vi "WriteCartesianPositionRegister.vi"(8 "Cartesian position":T1, 9 "index":i32, 10 "Snpx":refnum<k24>, 11 "error in":errorcluster) -> (3 "error out":errorcluster)   [LabVIEW 2016, in "UnderAutomation.Fanuc.lvlib"]
uses:
  UnderAutomation.Fanuc.lvlib
  C:/Users/fg/Documents/Fanuc.vi/LabVIEW_2024/UnderAutomation.Fanuc/lib/UnderAutomation.Fanuc.dll
  LabVIEW_2024/UnderAutomation.Fanuc/lib/UnderAutomation.Fanuc.dll
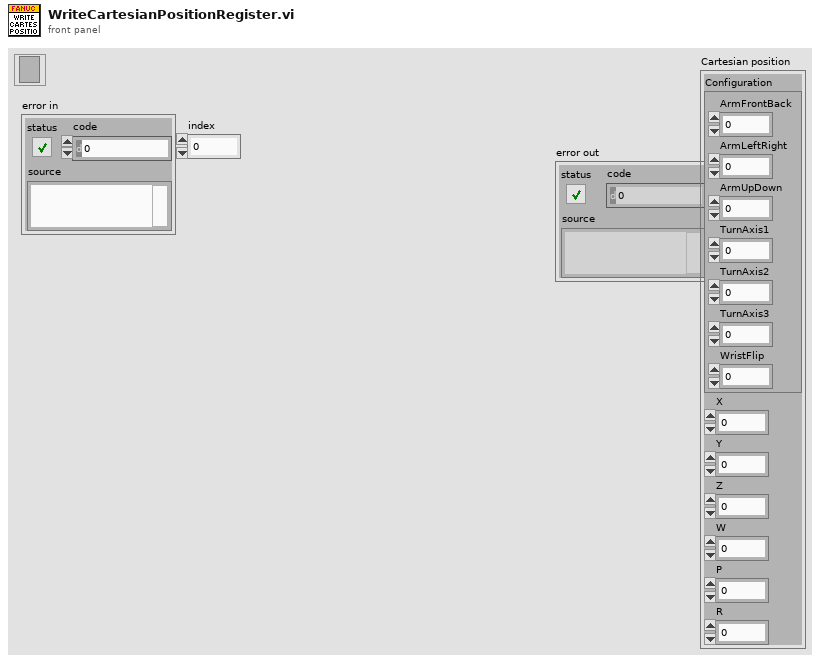
[diagram p1: front panel]
types:
  T1 = cluster{"Configuration":cluster{"ArmFrontBack":i32, "ArmLeftRight":i32, "ArmUpDown":i32, "TurnAxis1":i32, "TurnAxis2":i32, "TurnAxis3":i32, "WristFlip":i32}, "X":dbl, "Y":dbl, "Z":dbl, "W":dbl, "P":dbl, "R":dbl}
  T2 = cluster{"ArmFrontBack":i32, "ArmLeftRight":i32, "ArmUpDown":i32, "TurnAxis1":i32, "TurnAxis2":i32, "TurnAxis3":i32, "WristFlip":i32}
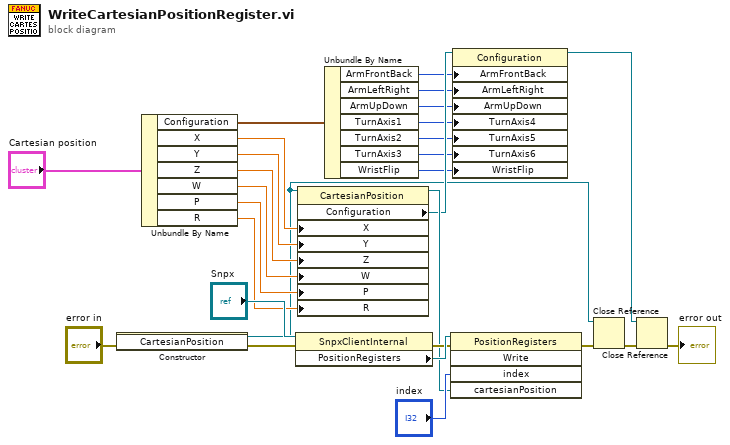
[diagram p0: block diagram]
diagram:
  n1 = constructor class="CartesianPosition"(error in="error in") -> (reference out=w4:refnum<k24>, error out=w6:errorcluster)  [unwired: 2 in, 1 out]
  n2 = Unbundle By Name("Cartesian position") -> ("Configuration"=w22:T2, "X"=w13:dbl, "Y"=w12:dbl, "Z"=w11:dbl, "W"=w10:dbl, "P"=w9:dbl, "R"=w8:dbl)
  n3 = property class="SnpxClientInternal"(reference="Snpx", error in=w6) -> (error out=w26:errorcluster, "PositionRegisters"=w27:refnum<k24>)  [unwired: 1 out]
  n4 = property class="CartesianPosition"(reference=w4, "X"=w13, "Y"=w12, "Z"=w11, "W"=w10, "P"=w9, "R"=w8) -> (reference out=w24:refnum<k24>, "Configuration"=w23:refnum<k24>)  [unwired: 1 in, 1 out]
  n5 = Unbundle By Name(w22) -> ("ArmFrontBack"=w21:i32, "ArmLeftRight"=w20:i32, "ArmUpDown"=w19:i32, "TurnAxis1"=w18:i32, "TurnAxis2"=w17:i32, "TurnAxis3"=w16:i32, "WristFlip"=w15:i32)
  n6 = invoke class="PositionRegisters" method="Write"(reference=w27, error in=w26, "index"="index", "cartesianPosition"=w24) -> (error out=w5:errorcluster)  [unwired: 1 in, 4 out]
  n7 = property class="Configuration"(reference=w23, "ArmFrontBack"=w21, "ArmLeftRight"=w20, "ArmUpDown"=w19, "TurnAxis4"=w18, "TurnAxis5"=w17, "TurnAxis6"=w16, "WristFlip"=w15) -> (reference out=w1:refnum<k24>)  [unwired: 1 in, 1 out]
  n8 = Close Reference(reference=w4, error in (no error)=w5) -> (error out=w3:errorcluster)
  n9 = Close Reference(reference=w1, error in (no error)=w3) -> (error out=→"error out":errorcluster)
